vi "OPM.SetWavelength.vi"(8 "error in (no error)":errorcluster, 10 "Wavelength, nm":dbl, 11 "OPM.ThorlabsPM400 in":refnum<class "OPM.ThorlabsPM400.lvclass">) -> (0 "error out":errorcluster, 3 "OPM.ThorlabsPM400 out":refnum<class "OPM.ThorlabsPM400.lvclass">)   [LabVIEW 2019, in "OPM.ThorlabsPM400.lvclass"]
uses:
  OPM.ThorlabsPM400.lvclass
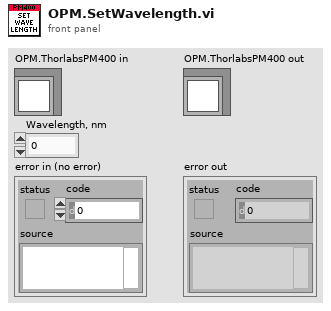
[diagram p1: front panel]
types:
  T1 = typedef "OPM.ThorlabsPM400.lvclass/Resource--Cluster.ctl" = cluster{"Instrument handle":refnum<visa-resource-name>}
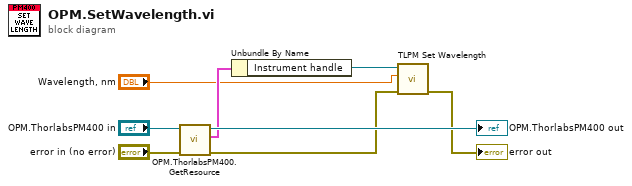
[diagram p0: block diagram]
diagram:
  n1 = call "OPM.ThorlabsPM400.GetResource.vi"("error in (no error)"="error in (no error)", "OPM.ThorlabsPM400 in"="OPM.ThorlabsPM400 in") -> ("error out"=w4:errorcluster, "Resource"=w5:T1, "OPM.ThorlabsPM400 out"=→"OPM.ThorlabsPM400 out":refnum<class "OPM.ThorlabsPM400.lvclass">)  [unwired: 7 in]
  n2 = Unbundle By Name(w5) -> ("Instrument handle"=w2:refnum<visa-resource-name>)
  n3 = call <instrlib>:"TLPM Set Wavelength.vi"("error in (no error)"=w4, "Wavelength (0.0)"="Wavelength, nm", "instrument handle"=w2) -> ("error out"=→"error out":errorcluster)  [unwired: 7 in, 1 out]
